vi "Exchange Command.vi"(6 "Synchronization":enum16{"Start", "Wait"}(ring), 7 "Description":string, 8 "Command Info In":T3) -> (0 "Command Info Out":T3)   [LabVIEW 2018]
doc: "This template has a parameter to control whether it waits for the command to complete or not. This is useful for operations that have a timed duration or a sensor-based duration. \n\nBe sure to right-click and select New from Template and save with a new command name."
uses:
  <vilib>/Rock Robotics/WPI/Framework/Command Status Info.ctl
  <vilib>/Rock Robotics/WPI/Framework/Completion Status.ctl
  <vilib>/Rock Robotics/WPI/Framework/Completion Notifier.ctl
  Implementation/Sequencer Type.ctl
  Implementation/All Commands.ctl
  Implementation/Subsystem Sequencer Setpoints.ctl
  Implementation/Subsystem Sequencer Operations.ctl
panel:
  in  "Sequence":T1[](array[typedef])=[{"Cmd"=enum."Elevator - Elevator Set Position Wait", "Value"=0.0}, {"Cmd"=enum."Arm - Arm to Pickup Position", "Value"=0.0}]
  # "Right click the ARRAY, Data Operation --> Set Current Values as Default"
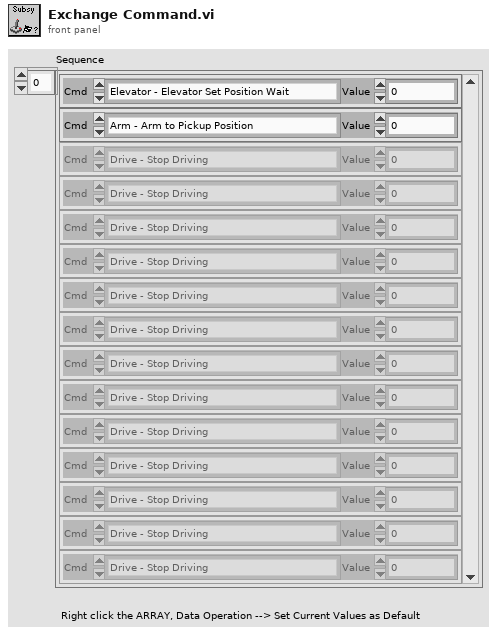
[diagram p1: front panel]
types:
  T1 = typedef "Sequencer Type.ctl" = cluster{"Cmd":T2, "Value":dbl}
  T2 = typedef "All Commands.ctl" = enum16{"Wait ms", "Drive - Stop Driving", "Drive - Drive Distance Straight", "Elevator - Elevator Stop", "Elevator - Elevator Set Position Wait", "Elevator - Elevator Set Position Start", "Arm - Arm to Shoot Position", "Arm - Arm to Pickup Position", "Arm - Arm Set Position"}
  T3 = typedef "Command Status Info.ctl" = cluster{"Name":string, "Status":T4, "notifier out":T5}
  T4 = typedef "Completion Status.ctl" = enum16{"Successful", "Aborted", "Incomplete"}
  T5 = typedef "Completion Notifier.ctl" = refnum<notifier>
  T6 = typedef "Subsystem Sequencer Setpoints.ctl" = cluster{"Operation":T7, "Setpoint":dbl, "Duration":dbl}
  T7 = typedef "Subsystem Sequencer Operations.ctl" = enum16{"Reserve", "Read Current", "Run Sequence"}
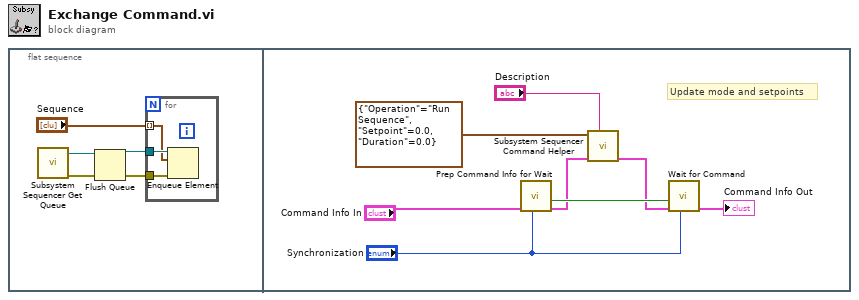
[diagram p0: block diagram]
diagram:
  n1 = flat-sequence {
    frame #0 {
      n2 = call "Subsystem Sequencer Get Queue.vi"() -> ("error out"=w3:errorcluster, "queue out"=w5:refnum<queue>)  [unwired: 10 in]
      n3 = Flush Queue(queue=w5, error in (no error)=w3) -> (queue out=w4:refnum<queue>, error out=w2:errorcluster)  [unwired: 1 out]
      n4 = for {
        tunnel: w4 -> [w8]
        tunnel: w2 -> [w7]
        tunnel: "Sequence" -> [w6] mode=indexing
        n5 = Enqueue Element(queue=w8, element=w6, error in (no error)=w7) -> ()  [unwired: 1 in, 3 out]
      }
    }
    frame #1 {
      # "Update mode and setpoints"
      n6 = call <vilib>:"Prep Command Info for Wait.vi"("Synchronication"="Synchronization", "Command Info"="Command Info In") -> ("Command Info"=w14:T3, "Allocated"=w15:bool)  [unwired: 8 in]
      n7 = call "Subsystem Sequencer Command Helper.vi"("Description"="Description", "Command Info In"=w14, "SubSystem Data"=T6 {"Operation"=enum."Run Sequence", "Setpoint"=0.0, "Duration"=0.0}) -> ("Command Info Out"=w11:T3)  [unwired: 6 in, 2 out]
      n8 = call <vilib>:"Wait for Command.vi"("Synchronication"="Synchronization", "Command Info in"=w11, "Allocated"=w15) -> ("Command Info out"=→"Command Info Out":T3)  [unwired: 8 in]
    }
  }
